vi "test-PID-test-02-RotateToTarget.vi"() -> (3 "All Passed":bool)   [LabVIEW 2019]
uses:
  <vilib>/Rock Robotics/WPI/ThirdParty/JAS_Junk/TrajLib/ControllerUtil_GetModulusError.vi
  <vilib>/Rock Robotics/WPI/ThirdParty/JAS_Junk/TrajLib/Trajectory_Library.lvlib
panel:
  out "Waveform Chart":cluster{"ControlOutput":dbl, dbl}(graph)
  out "Position":dbl
  out "ControlOutput":dbl
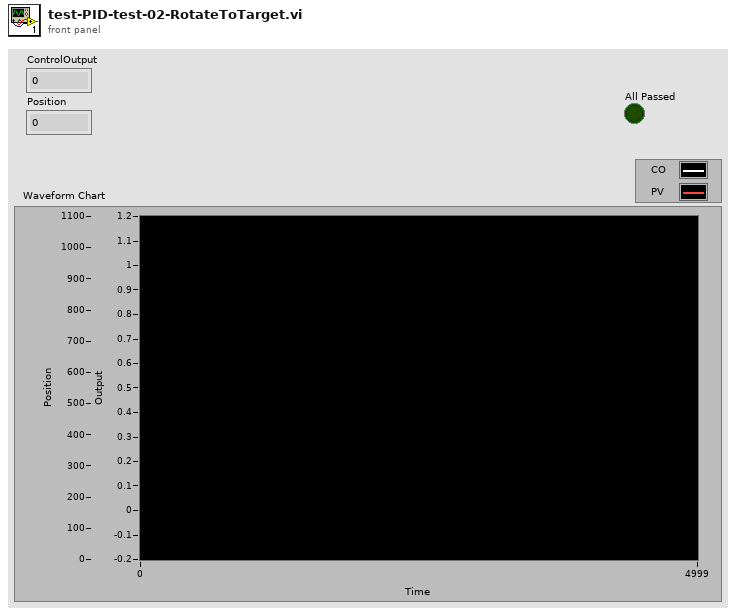
[diagram p1: front panel]
types:
  T1 = typedef "Trajectory_Library.lvlib/PID_CONTROLLER.ctl" = cluster{"Kp":dbl, "Ki":dbl, "Kd":dbl, "Period":dbl, "Max_Integral":dbl, "Min_Integral":dbl, "Max_Input":dbl, "Min_Input":dbl, "Continuous":bool, "PositionError":dbl, "VelocityError":dbl, "PrevError":dbl, "TotalError":dbl, "PositionTolerance":dbl, "VelocityTolerance":dbl, "SetPoint":dbl, "Kf":dbl, "Prev_Deriv":dbl, "Prev_Deriv 2":dbl, "DerivativeFilter":bool, "Min_Output":dbl, "Max_Output":dbl, "Prev_F_P":dbl, "Prev_F_P_2":dbl, "AntiWindupActive":bool, "Measurement":dbl}
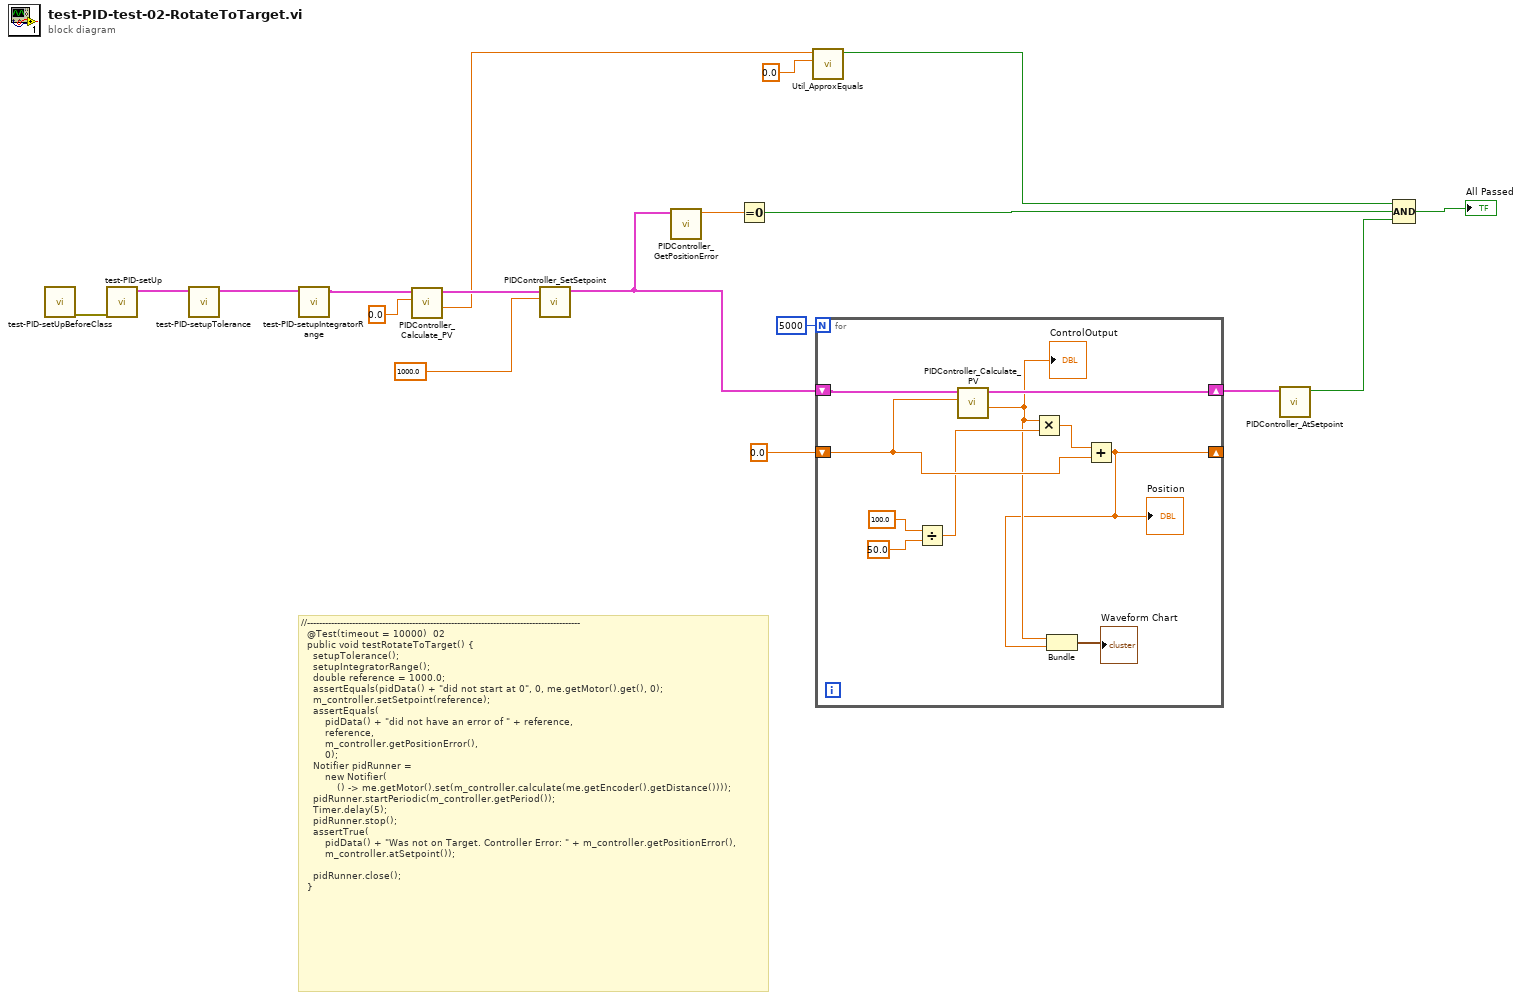
[diagram p0: block diagram]
diagram:
  # "//-------------------------------------------------------------------------------------------\n  @Test(timeout = 10000)  02\n  public void testRotateToTarget() {\n    setupTolerance();\n    setupIntegratorRange();\n    double reference = 1000.0;\n    assertEquals(pidData() + \"did not start at 0\", 0, me.getMotor().get(), 0);\n    m_controller.setSetpoint(reference);\n    assertEquals(\n        pidData() + \"did not have an error of \" + reference,\n        reference,\n        m_controller.getPositionError(),\n        0);\n    Notifier pidRunner =\n        new Notifier(\n            () -> me.getMotor().set(m_controller.calculate(me.getEncoder().getDistance())));\n    pidRunner.startPeriodic(m_controller.getPeriod());\n    Timer.delay(5);\n    pidRunner.stop();\n    assertTrue(\n        pidData() + \"Was not on Target. Controller Error: \" + m_controller.getPositionError(),\n        m_controller.atSetpoint());\n\n    pidRunner.close();\n  }"
  n1 = call "test-PID-setUpBeforeClass.vi"() -> ("error out"=w18:errorcluster)  [unwired: 11 in]
  n2 = call "test-PID-setUp.vi"("error in (no error)"=w18) -> ("PID_CONTROLLER"=w17:T1)  [unwired: 9 in, 1 out]
  n3 = call "test-PID-setupTolerance.vi"("in PID_CONTROLLER"=w17) -> ("out PID_CONTROLLER"=w16:T1)  [unwired: 10 in]
  n4 = call "test-PID-setupIntegratorRange.vi"("in PID_CONTROLLER"=w16) -> ("out PID_CONTROLLER"=w12:T1)  [unwired: 10 in]
  n5 = call <vilib>:"PIDController_Calculate_PV.vi"("PV"=0.0, "in PID_CONTROLLER"=w12) -> ("ControlOutput"=w10:dbl, "out PID_CONTROLLER"=w11:T1)  [unwired: 8 in]
  n6 = call <vilib>:"PIDController_SetSetpoint.vi"("Setpoint"=1000.0, "in PID_CONTROLLER"=w11) -> ("out PID_CONTROLLER"=w5:T1)  [unwired: 9 in]
  n7 = call <vilib>:"PIDController_GetPositionError.vi"("in PID_CONTROLLER"=w5) -> ("PositionError"=w15:dbl)  [unwired: 10 in]
  n8 = Equal To 0?(x=w15) -> (x = 0?=w6:bool)
  n9 = call <vilib>:"Util_ApproxEquals.vi"("Value 2"=0.0, "Value 1"=w10) -> ("ApproxEquals"=w8:bool)  [unwired: 9 in]
  n10 = for {
    N: 5000 -> [_]
    shift-right: [w28] -> w2
    shift-left: w5 -> [w27]
    shift-right: [w20] -> _
    shift-left: 0.0 -> [w25]
    n11 = Divide(x=100.0, y=50.0) -> (x/y=w22:dbl)
    n12 = call <vilib>:"PIDController_Calculate_PV.vi"("PV"=w25, "in PID_CONTROLLER"=w27) -> ("ControlOutput"=w21:dbl, "out PID_CONTROLLER"=w28:T1)  [unwired: 8 in]
    "ControlOutput" <- w21
    n13 = Multiply(x=w21, y=w22) -> (x*y=w26:dbl)
    n14 = Add(x=w26, y=w25) -> (x+y=w20:dbl)
    "Position" <- w20
    n15 = Bundle("ControlOutput"=w21, w20) -> (→"Waveform Chart":cluster{"ControlOutput":dbl, dbl})  [unwired: 1 in]
  }
  n16 = call <vilib>:"PIDController_AtSetpoint.vi"("in PID_CONTROLLER"=w2) -> ("AtSetpoint"=w1:bool)  [unwired: 10 in]
  n17 = Compound Arithmetic op=AND(w8, w6, w1) -> (→"All Passed":bool)
